vi "InTake Process.vi"(0 "error in":errorcluster) -> ()   [LabVIEW 2013]
uses:
  InTake Global Data.vi
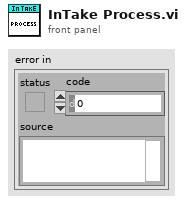
[diagram p1: front panel]
types:
  T1 = cluster{"TakeBall":dbl, "UpperClaw":dbl, "LowerClaw":dbl, "MS":bool, "Upper claw max":bool, "Lower claw max":bool, "Upper claw min":bool, "Lower claw min":bool, "Angle":dbl}
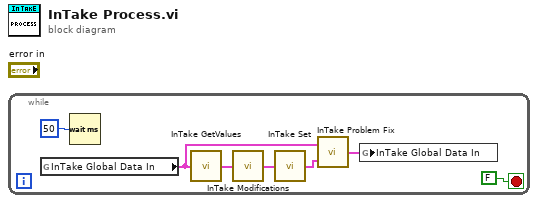
[diagram p0: block diagram]
diagram:
  n1 = while {
    stop <- FALSE stop-if-true
    n2 = global read "InTake Global Data.vi" "InTake Global Data In"() -> (w1:T1)
    n3 = Wait (ms)(milliseconds to wait=u32 50) -> ()  [unwired: 1 out]
    n4 = call "InTake GetValues.vi"("InTake Global Data In"=w1) -> ("InTake Global Data Out"=w5:T1)
    n5 = call "InTake Modifications.vi"("InTake Global Data In"=w5) -> ("InTake Global Data Out"=w4:T1)
    n6 = call "InTake Set.vi"("InTake Global Data In"=w4) -> ("InTake Global Data Out"=w3:T1)
    n7 = call "InTake Problem Fix.vi"("InTake Global Data Modified"=w3, "InTake Global Data Original"=w1) -> ("InTake Global Data New"=w2:T1)
    n8 = global write "InTake Global Data.vi" "InTake Global Data In"(w2) -> ()
  }
